vi "Pack Write Request.vi"(9 "Execution Callback":refnum<class "IWriteExecutionCallback.lvclass">, 10 "Packet":refnum<class "IPacket.lvclass">, 11 "WriteRequest in":refnum<class "WriteRequest.lvclass">) -> (3 "WriteRequest out":refnum<class "WriteRequest.lvclass">)   [LabVIEW 2019, in "MessagingInterfaces.lvlib" / "WriteRequest.lvclass"]
uses:
  <vilib>/gpm_packages/@cs/Network-interface/Source/MessagingInterfaces/WriteRequest/WriteRequest.lvclass
  <vilib>/gpm_packages/@cs/Network-interface/Source/MessagingInterfaces/IWriteExecutionCallback/IWriteExecutionCallback.lvclass
  <vilib>/gpm_packages/@cs/Network-interface/Source/MessagingInterfaces/IPacket/IPacket.lvclass
  <vilib>/gpm_packages/@cs/Network-interface/Source/MessagingInterfaces/WriteRequest/WriteRequest.lvclass/WriteRequest.ctl
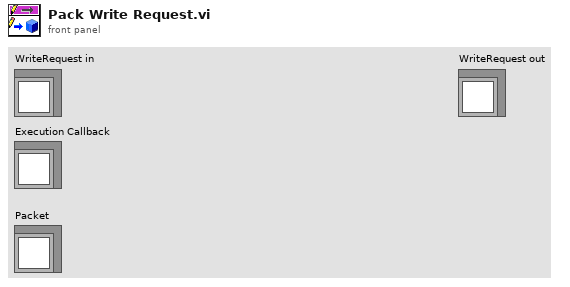
[diagram p1: front panel]
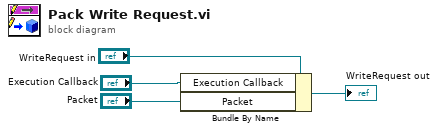
[diagram p0: block diagram]
diagram:
  n1 = Bundle By Name(cluster="WriteRequest in", "Execution Callback"="Execution Callback", "Packet"="Packet") -> (→"WriteRequest out":refnum<class "WriteRequest.lvclass">)
